vi "Stop Calibration.vi"(8 "Error in (no error)":errorcluster, 11 "VISA resource name":refnum<visa-resource-name>) -> (0 "Error out":errorcluster, 3 "VISA resource name out":refnum<visa-resource-name>)   [LabVIEW 2011, in "Ocean Server OS4000.lvlib"]
doc: "Sends Command to Instrument to stop calibrating"
uses:
  Ocean Server OS4000.lvlib
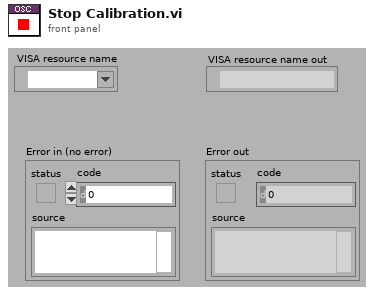
[diagram p1: front panel]
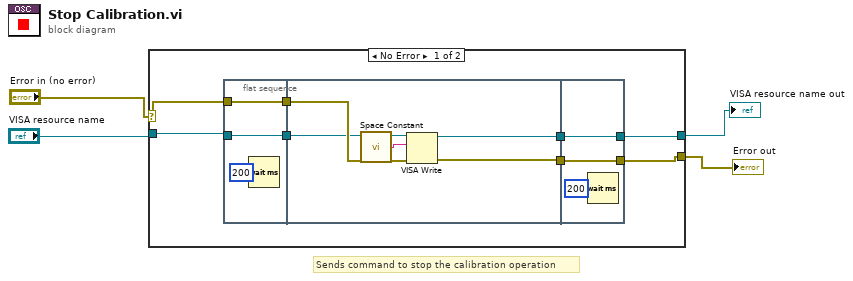
[diagram p0: block diagram]
diagram:
  # "Sends command to stop the calibration operation"
  n1 = case shown="No Error" "Error in (no error)" {
    selector: "Error in (no error)" -> [w12 w25]
    tunnel: "VISA resource name" -> [w11 w24]
    tunnel: [w5 w25] -> w2
    tunnel: [w7 w24] -> w1
    frame No Error {
      n2 = flat-sequence {
        tunnel: w11 -> [w14]
        tunnel: w12 -> [w15]
        tunnel: [w15] -> w10
        tunnel: [w14] -> w9
        tunnel: w10 -> [w20]
        tunnel: w9 -> [w19]
        tunnel: [w18] -> w8
        tunnel: [w16] -> w6
        tunnel: [w23] -> w5
        tunnel: w8 -> [w23]
        tunnel: [w21] -> w7
        tunnel: w6 -> [w21]
        frame #0 {
          n3 = Wait (ms)(milliseconds to wait=u32 200) -> ()  [unwired: 1 out]
        }
        frame #1 {
          n4 = call <vilib>:"Space Constant.vi"() -> ("String"=w17:string)
          n5 = VISA Write(VISA resource name=w19, write buffer=w17, error in (no error)=w20) -> (VISA resource name out=w16:refnum<visa-resource-name>, error out=w18:errorcluster)  [unwired: 1 out]
        }
        frame #2 {
          n6 = Wait (ms)(milliseconds to wait=u32 200) -> ()  [unwired: 1 out]
        }
      }
    }
    frame Error {
    }
  }
  "Error out" <- w2
  "VISA resource name out" <- w1
